vi "verify acquisition progress.vi"(8 "error in (no error)":errorcluster, 11 "SPARC4_Channel in":refnum<class "SPARC4_Channel.lvclass">) -> (0 "error out":errorcluster, 2 "acq in progress":T1, 3 "SPARC4_Channel out":refnum<class "SPARC4_Channel.lvclass">)   [LabVIEW 2018, in "SPARC4_Channel.lvclass"]
uses:
  SPARC4_Channel.lvclass
  SPARC4_Channel.lvclass/SPARC4_Channel.ctl
  Sim_CCD/Sim_CCD.lvclass
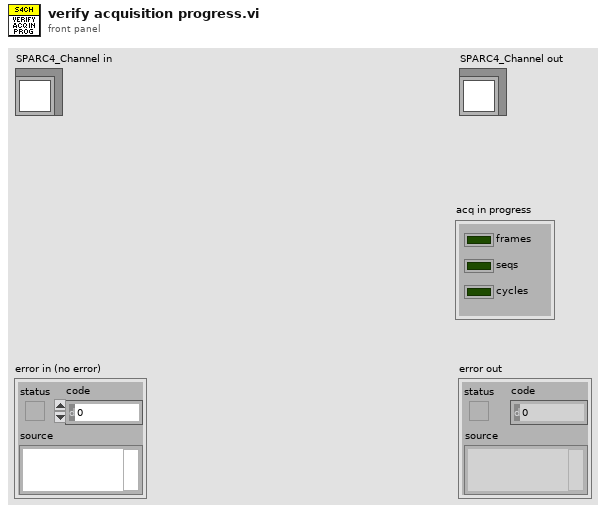
[diagram p1: front panel]
types:
  T1 = cluster{"frames":bool, "seqs":bool, "cycles":bool}
  T2 = cluster{"CYCLES_DONE":u16, "LAST_IMAGE_NAME":string, "USED_DISK_SPACE":u16, "IMAGE_INDEX":u32, "acquisition error":bool}
  T3 = cluster{"SEQS_DONE":u16, "S4ICS comm attempts":u8}
  T4 = cluster{"State Machine.lvclass":refnum<class "State Machine.lvclass">, "RxTx.lvclass":refnum<class "RxTx.lvclass">, "Save_Header_RxTx.lvclass":refnum<class "RxTx.lvclass">, "Status SM.lvclass":refnum<class "State Machine.lvclass">, "Status RxTx.lvclass":refnum<class "RxTx.lvclass">, "servers array":refnum<class "Server.lvclass">[], "Events log file.lvclass":refnum<class "Log File.lvclass">, "Errors log file.lvclass":refnum<class "Log File.lvclass">, "Keywords log file.lvclass":refnum<class "Log File.lvclass">, "Sim_CCD.lvclass":refnum<class "Sim_CCD.lvclass">}
  T5 = cluster{"FRAMES_DONE":u16, "CCD_STATUS":string, "CURRENT_TEMPERATURE":i16, "TEMPERATURE_STATUS":string, "FRAME_EXPOSURE_TIME":sgl, "SERIAL_NUMBER":u16, "ACQUIRING":bool, "POWER":bool}
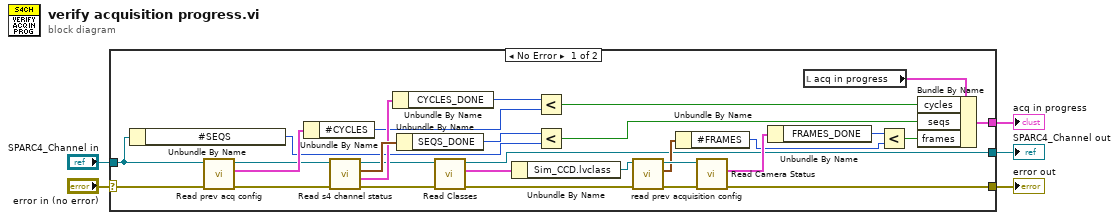
[diagram p0: block diagram]
diagram:
  n1 = case shown="No Error" "error in (no error)" {
    selector: "error in (no error)" -> [w29 w36]
    tunnel: [w18 w36] -> w4
    tunnel: [w17 w35] -> w2
    tunnel: "SPARC4_Channel in" -> [w28 w35]
    tunnel: [w13 _] -> w1
    frame No Error {
      n2 = Unbundle By Name(w28) -> ("#SEQS"=w10:u32)
      n3 = call-dynamic "Read prev acq config.vi"("error in (no error)"=w29, "Channel in"=w28) -> ("error out"=w31:errorcluster, "prev acq config"=w34:cluster{"suffix":string, "#CYCLES":u32}, "Channel out"=w30:refnum<class "SPARC4_Channel.lvclass">)  [unwired: 7 in]
      n4 = Unbundle By Name(w34) -> ("#CYCLES"=w15:u32)
      n5 = call "Read s4 channel status.vi"("error in (no error)"=w31, "SPARC4_Channel in"=w30) -> ("error out"=w26:errorcluster, "channel status"=w32:T2, "s4 channel status"=w33:T3, "SPARC4_Channel out"=w27:refnum<class "SPARC4_Channel.lvclass">)  [unwired: 6 in]
      n6 = Unbundle By Name(w32) -> ("CYCLES_DONE"=w16:u16)
      n7 = Unbundle By Name(w33) -> ("SEQS_DONE"=w11:u16)
      n8 = call-dynamic "Read Classes.vi"("error in (no error)"=w26, "Channel in"=w27) -> ("error out"=w21:errorcluster, "Classes"=w25:T4, "Channel out"=w17:refnum<class "SPARC4_Channel.lvclass">)  [unwired: 7 in]
      n9 = Unbundle By Name(w25) -> ("Sim_CCD.lvclass"=w23:refnum<class "Sim_CCD.lvclass">)
      n10 = Less?(x=w16, y=w15) -> (x < y?=w12:bool)
      n11 = Less?(x=w11, y=w10) -> (x < y?=w9:bool)
      n12 = call "read prev acquisition config.vi"("error in (no error)"=w21, "Simulated_CCD_Camera in"=w23) -> ("error out"=w20:errorcluster, "Prev SET parameters"=w19:cluster{"EXPTIME":dbl, "#FRAMES":u32}, "Simulated_CCD_Camera out"=w22:refnum<class "Sim_CCD.lvclass">)  [unwired: 7 in]
      n13 = Unbundle By Name(w19) -> ("#FRAMES"=w6:u32)
      n14 = call "Read Camera Status.vi"("error in (no error)"=w20, "CCDCamera in"=w22) -> ("error out"=w18:errorcluster, "camera status"=w24:T5)  [unwired: 7 in, 1 out]
      n15 = Unbundle By Name(w24) -> ("FRAMES_DONE"=w7:u16)
      n16 = local read "acq in progress"() -> (w14:T1)
      n17 = Less?(x=w7, y=w6) -> (x < y?=w8:bool)
      n18 = Bundle By Name(cluster=w14, "cycles"=w12, "seqs"=w9, "frames"=w8) -> (w13:T1)
    }
    frame Error {
    }
  }
  "error out" <- w4
  "SPARC4_Channel out" <- w2
  "acq in progress" <- w1
